vi "Speed Mode.vi"(8 "error in (no error)":errorcluster, 10 "String":string, 11 "Low Speed in":refnum<class "Low Speed.lvclass">) -> (0 "error out 2":errorcluster, 2 "This VI":refnum<vi>, 3 "Low Speed out":refnum<class "Low Speed.lvclass">)   [LabVIEW 2020, in "Low Speed.lvclass"]
uses:
  Low Speed.lvclass
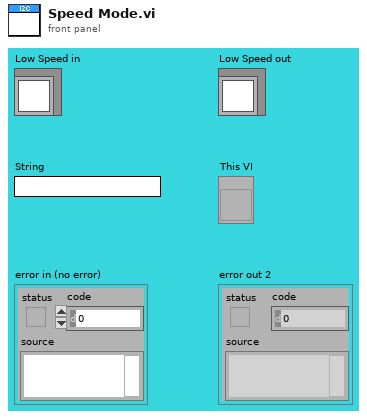
[diagram p1: front panel]
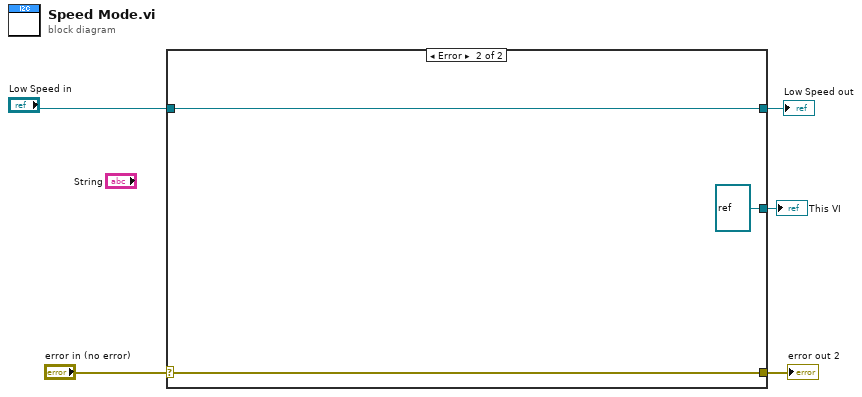
[diagram p0: block diagram]
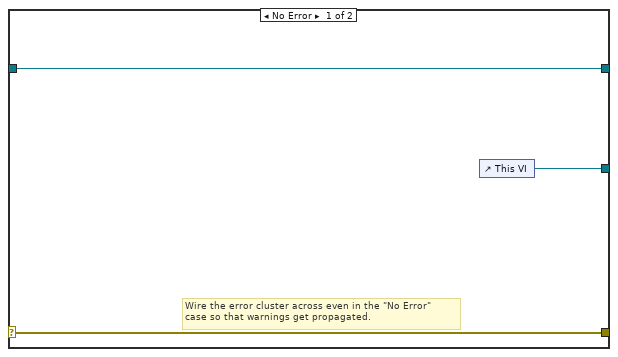
[diagram p2: hidden frame]
diagram:
  n1 = case shown="Error" "error in (no error)" {
    selector: "error in (no error)" -> [w7 w11]
    tunnel: [w7 w11] -> w4
    tunnel: [w8 w10] -> w1
    tunnel: "Low Speed in" -> [w8 w10]
    tunnel: [w6 refnum<vi> refnum ("This VI")] -> w3
    frame No Error {
      # "Wire the error cluster across even in the \"No Error\"\ncase so that warnings get propagated."
      n2 = control-ref of="This VI"() -> (w6:refnum<vi>)
    }
    frame Error {
    }
  }
  "Low Speed out" <- w1
  "error out 2" <- w4
  "This VI" <- w3
